vi "DepthSense Connect Callback 2.vi"(4 "User Parameter":variant, 6 "Control Ref":refnum<k24>, 7 "Event Common Data":T1) -> ()   [LabVIEW 2011]
uses:
  C:/Users/Behavior Room/Desktop/Kinect Mouse/DepthSense/FunctionPointerProxy/FunctionPointerProxy/bin/Release/FunctionPointerProxy.dll
  FunctionPointerProxy/FunctionPointerProxy/bin/Release/FunctionPointerProxy.dll
  DepthSense Global Status.vi
  <userlib>/libOptrima-2-3/libOptrima-2-3.lvlib
panel:
  out "error out":errorcluster
  out "camera version":string
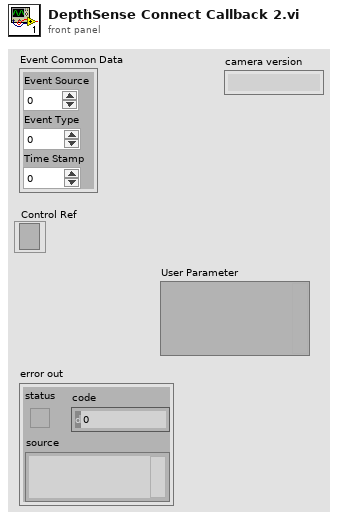
[diagram p1: front panel]
types:
  T1 = cluster{"Event Source":i32, "Event Type":u32, "Time Stamp":u32}
  T2 = typedef "DepthSense State.ctl" = cluster{"Camera Version":string, "Image Height":i32, "Image Width":i32, "Minimum Framerate":i32, "Maximum Framerate":i32, "Framerate":i32, "Close Mode":bool, "Denoising":bool, "Leakage Algorithm":bool, "Anti-Aliasing":bool, "Camera Status":i32, "API Version":string, "Light Intensity":i32}
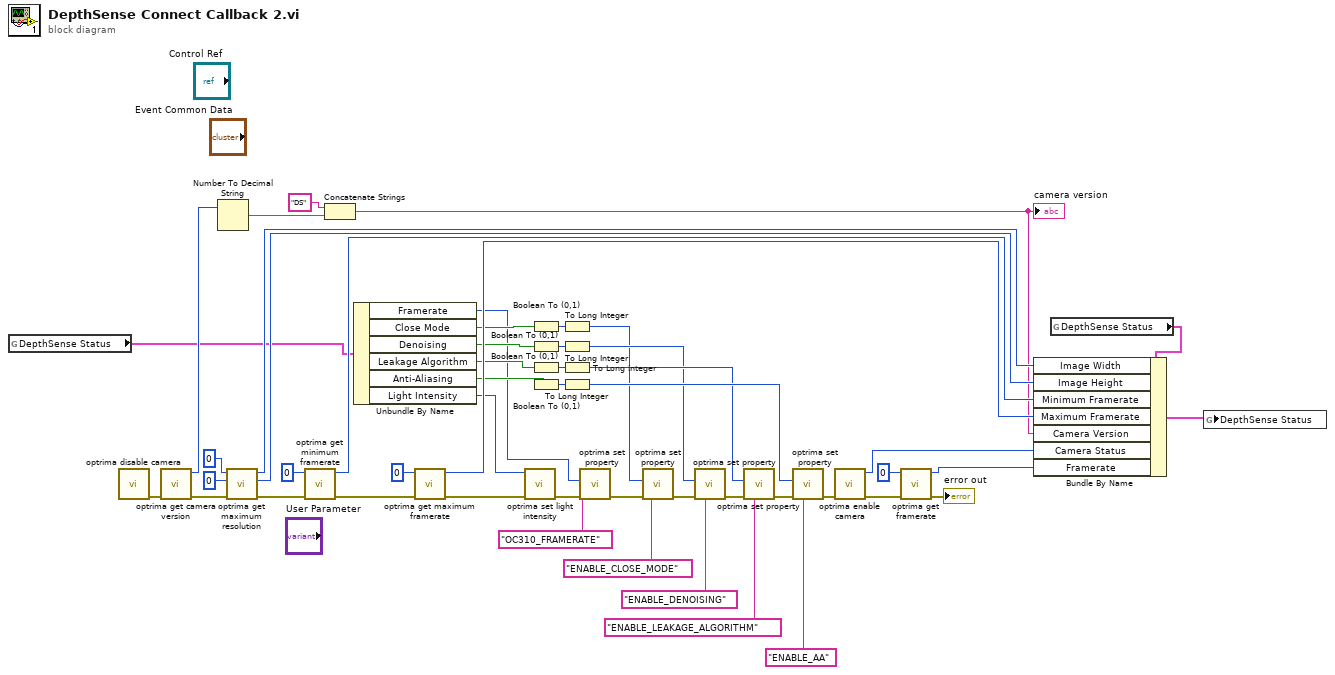
[diagram p0: block diagram]
diagram:
  n1 = global read "DepthSense Global Status.vi" "DepthSense Status"() -> (w7:T2)
  n2 = call <userlib>:"optrima disable camera.vi"() -> ("error out"=w50:errorcluster)  [unwired: 10 in, 1 out]
  n3 = call <userlib>:"optrima get camera version.vi"("error in (no error)"=w50) -> ("error out"=w38:errorcluster, "version out"=w49:u32)  [unwired: 8 in, 1 out]
  n4 = Number To Decimal String(number=w49) -> (decimal integer string=w48:string)  [unwired: 1 in]
  n5 = call <userlib>:"optrima get maximum resolution.vi"("error in (no error)"=w38, "rows"=u32 0, "columns"=u32 0) -> ("error out"=w44:errorcluster, "rows out"=w27:u32, "columns out"=w28:u32)  [unwired: 5 in, 1 out]
  n6 = call <userlib>:"optrima get minimum framerate.vi"("error in (no error)"=w44, "min_framerate"=u32 0) -> ("error out"=w42:errorcluster, "min_framerate out"=w26:u32)  [unwired: 7 in, 1 out]
  n7 = Concatenate Strings("DS" ("string"), w48) -> (w24:string)
  "camera version" <- w24
  n8 = Unbundle By Name(w7) -> ("Framerate"=w10:i32, "Close Mode"=w23:bool, "Denoising"=w22:bool, "Leakage Algorithm"=w21:bool, "Anti-Aliasing"=w20:bool, "Light Intensity"=w11:i32)
  n9 = call <userlib>:"optrima get maximum framerate.vi"("error in (no error)"=w42, "max_framerate"=u32 0) -> ("error out"=w15:errorcluster, "max_framerate out"=w25:u32)  [unwired: 7 in, 1 out]
  n10 = call <userlib>:"optrima set light intensity.vi"("error in (no error)"=w15, "intensity_percentage"=w11) -> ("error out"=w40:errorcluster)  [unwired: 8 in, 1 out]
  n11 = Boolean To (0,1)(Boolean=w23) -> (0, 1=w19:i16)
  n12 = Boolean To (0,1)(Boolean=w22) -> (0, 1=w18:i16)
  n13 = Boolean To (0,1)(Boolean=w21) -> (0, 1=w17:i16)
  n14 = Boolean To (0,1)(Boolean=w20) -> (0, 1=w16:i16)
  n15 = To Long Integer(number=w19) -> (32bit integer=w1:i32)
  n16 = To Long Integer(number=w18) -> (32bit integer=w2:i32)
  n17 = To Long Integer(number=w17) -> (32bit integer=w3:i32)
  n18 = To Long Integer(number=w16) -> (32bit integer=w4:i32)
  n19 = call <userlib>:"optrima set property.vi"("error in (no error)"=w40, "value"=w10, "name"="OC310_FRAMERATE") -> ("error out"=w37:errorcluster)  [unwired: 7 in, 1 out]
  n20 = call <userlib>:"optrima set property.vi"("error in (no error)"=w37, "value"=w1, "name"="ENABLE_CLOSE_MODE") -> ("error out"=w33:errorcluster)  [unwired: 7 in, 1 out]
  n21 = call <userlib>:"optrima set property.vi"("error in (no error)"=w33, "value"=w2, "name"="ENABLE_DENOISING") -> ("error out"=w32:errorcluster)  [unwired: 7 in, 1 out]
  n22 = call <userlib>:"optrima set property.vi"("error in (no error)"=w32, "value"=w3, "name"="ENABLE_LEAKAGE_ALGORITHM") -> ("error out"=w31:errorcluster)  [unwired: 7 in, 1 out]
  n23 = call <userlib>:"optrima set property.vi"("error in (no error)"=w31, "value"=w4, "name"="ENABLE_AA") -> ("error out"=w36:errorcluster)  [unwired: 7 in, 1 out]
  n24 = call <userlib>:"optrima enable camera.vi"("error in (no error)"=w36) -> ("error out"=w13:errorcluster, "function return"=w9:u32)  [unwired: 9 in]
  n25 = call <userlib>:"optrima get framerate.vi"("error in (no error)"=w13, "framerate"=u32 0) -> ("error out"=→"error out":errorcluster, "framerate out"=w8:u32)  [unwired: 7 in, 1 out]
  n26 = global read "DepthSense Global Status.vi" "DepthSense Status"() -> (w5:T2)
  n27 = Bundle By Name(cluster=w5, "Image Width"=w28, "Image Height"=w27, "Minimum Framerate"=w26, "Maximum Framerate"=w25, "Camera Version"=w24, "Camera Status"=w9, "Framerate"=w8) -> (w6:T2)
  n28 = global write "DepthSense Global Status.vi" "DepthSense Status"(w6) -> ()
